vi "move_tilt_stage_simple(Sub VI).vi"() -> ()   [LabVIEW 2016]
panel:
  out "Loop idx":i32
  out "open error":errorcluster
  out "Position":i32
  out "error out":errorcluster
  in  "stop":bool
  out "DeviceKey List Out":string[](array[string])
  in  "Num repeats":i32
  out "close error":errorcluster
  in  "Relative Steps":i32
  in  "Motor":i32
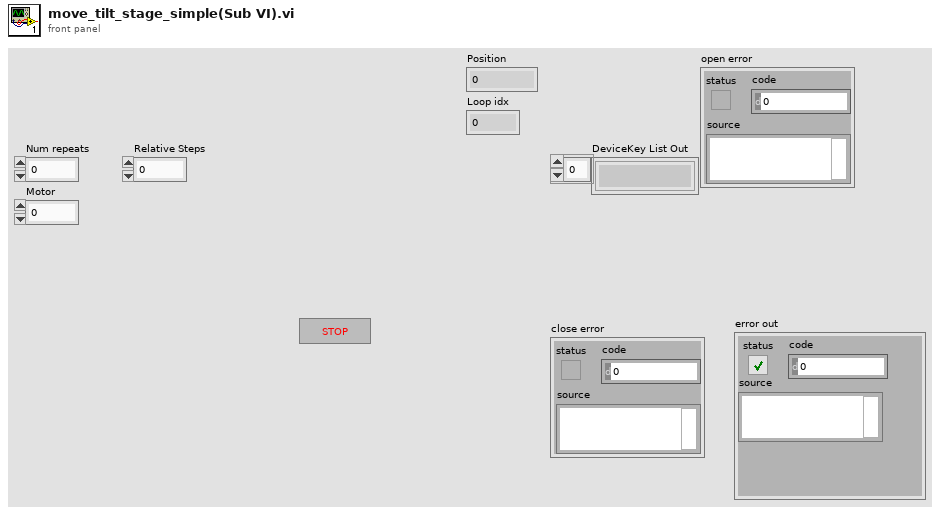
[diagram p1: front panel]
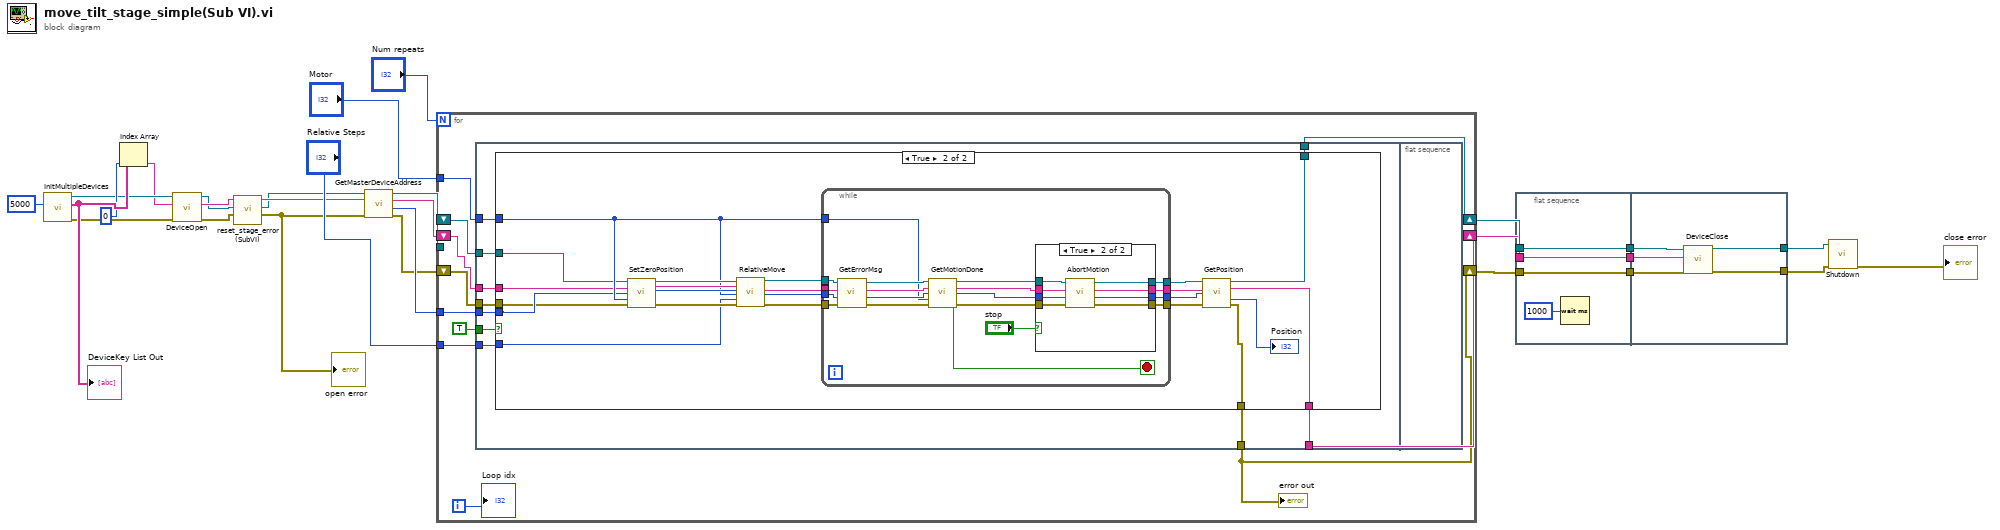
[diagram p0: block diagram]
diagram:
  n1 = call "InitMultipleDevices.vi"("msecDelayForDiscovery"=5000) -> ("error out"=w7:errorcluster, "DeviceKey List Out"=w25:string[], "CmdLib Out"=w9:refnum<k24>)  [unwired: 4 in]
  "DeviceKey List Out" <- w25
  n2 = Index Array(array=w25, index=0) -> (element=w8:string)
  n3 = call "DeviceOpen.vi"("error in (no error)"=w7, "DeviceKey In"=w8, "CmdLib In"=w9) -> ("error out"=w4:errorcluster, "DeviceKey Out"=w6:string, "CmdLib Out"=w5:refnum<k24>)  [unwired: 2 in]
  n4 = call "reset_stage_error (SubVI).vi"("error IO"=w4, "reference"=w5, "deviceKey"=w6) -> ("error IO 2"=w1:errorcluster, "new reference"=w2:refnum<k24>, "String"=w3:string)  [unwired: 6 in]
  "open error" <- w1
  n5 = call "GetMasterDeviceAddress.vi"("error in (no error)"=w1, "DeviceKey In"=w3, "CmdLib In"=w2) -> ("error out"=w19:errorcluster, "Device Address"=w20:i32, "DeviceKey Out"=w10:string, "CmdLib Out"=w21:refnum<k24>)  [unwired: 1 in]
  n6 = for {
    N: "Num repeats" -> [_]
    tunnel: "Motor" -> [w39]
    tunnel: w20 -> [w38]
    tunnel: "Relative Steps" -> [w35]
    shift-right: [w32] -> w15
    shift-left: w19 -> [w37]
    tunnel: w21 -> [_]
    shift-right: [w33] -> w16
    shift-left: w10 -> [w29]
    shift-right: [w34] -> w17
    shift-left: _ -> [w30]
    i -> [w31]
    n7 = flat-sequence {
      tunnel: w39 -> [w49]
      tunnel: w30 -> [w48]
      tunnel: w29 -> [w47]
      tunnel: [w44] -> _
      tunnel: TRUE ("Run?") -> [w46]
      tunnel: w35 -> [w45]
      tunnel: w38 -> [w44]
      tunnel: w37 -> [w43]
      tunnel: [w42] -> w34
      tunnel: [w41] -> w33
      tunnel: [w40] -> w32
      frame #0 {
        n8 = case shown="True" w46 {
          tunnel: w49 -> [_ w62]
          tunnel: w48 -> [w51 w61]
          tunnel: w47 -> [w52 w60]
          tunnel: w44 -> [_ w59]
          tunnel: w45 -> [_ w58]
          tunnel: w43 -> [w50 w57]
          tunnel: [w51 w56] -> w42
          tunnel: [w52 w55] -> w41
          tunnel: [w50 w54] -> w40
          frame False {
          }
          frame True {
            n9 = call "SetZeroPosition.vi"("CmdLib In"=w61, "DeviceKey In"=w60, "Device Address In"=w59, "Motor"=w62, "error in (no error)"=w57) -> ("CmdLib Out"=w71:refnum<k24>, "DeviceKey Out"=w70:string, "Device Address Out"=w68:i32, "error out"=w69:errorcluster)  [unwired: 7 in]
            n10 = call "RelativeMove.vi"("CmdLib In"=w71, "DeviceKey In"=w70, "Device Address In"=w68, "Motor"=w62, "Relative Steps"=w58, "error in (no error)"=w69) -> ("CmdLib Out"=w74:refnum<k24>, "DeviceKey Out"=w73:string, "Device Address Out"=w67:i32, "error out"=w72:errorcluster)  [unwired: 10 in]
            n11 = while {
              tunnel: w62 -> [w78]
              tunnel: w74 -> [w91]
              tunnel: w73 -> [w90]
              tunnel: [w86] -> w65
              tunnel: w67 -> [w85]
              tunnel: w72 -> [w89]
              tunnel: [w87] -> w66
              tunnel: [w77] -> w64
              tunnel: [w76] -> w63
              stop <- w83 stop-if-true
              n12 = call "GetErrorMsg.vi"("error in (no error)"=w89, "Device Address In"=w85, "DeviceKey In"=w90, "CmdLib In"=w91) -> ("error out"=w88:errorcluster, "Device Address Out"=w84:i32, "DeviceKey Out"=w93:string, "CmdLib Out"=w92:refnum<k24>)
              n13 = call "GetMotionDone.vi"("CmdLib In"=w92, "DeviceKey In"=w93, "Device Address In"=w84, "Motor"=w78, "error in (no error)"=w88) -> ("CmdLib Out"=w82:refnum<k24>, "DeviceKey Out"=w81:string, "Device Address Out"=w80:i32, "Is Motion Done"=w83:bool, "error out"=w79:errorcluster)  [unwired: 6 in]
              n14 = case shown="True" "stop" {
                tunnel: w79 -> [w96 w105]
                tunnel: [w96 w104] -> w87
                tunnel: w82 -> [w97 w103]
                tunnel: [w97 w102] -> w86
                tunnel: w81 -> [w94 w101]
                tunnel: w80 -> [w95 w100]
                tunnel: [w95 w99] -> w77
                tunnel: [w94 w98] -> w76
                frame False {
                }
                frame True {
                  n15 = call "AbortMotion.vi"("error in (no error)"=w105, "Device Address In"=w100, "DeviceKey In"=w101, "CmdLib In"=w103) -> ("error out"=w104:errorcluster, "Device Address Out"=w99:i32, "DeviceKey Out"=w98:string, "CmdLib Out"=w102:refnum<k24>)
                }
              }
            }
            n16 = call "GetPosition.vi"("CmdLib In"=w65, "DeviceKey In"=w63, "Device Address In"=w64, "error in (no error)"=w66) -> ("CmdLib Out"=w56:refnum<k24>, "DeviceKey Out"=w55:string, "Position"=→"Position":i32, "error out"=w54:errorcluster)  [unwired: 7 in, 1 out]
          }
        }
      }
      frame #1 {
      }
    }
    "error out" <- w32
    "Loop idx" <- w31
  }
  n17 = flat-sequence {
    tunnel: w15 -> [w107]
    tunnel: w16 -> [w108]
    tunnel: w17 -> [w109]
    tunnel: [w109] -> w28
    tunnel: [w108] -> w27
    tunnel: [w107] -> w26
    tunnel: w28 -> [w114]
    tunnel: w27 -> [w113]
    tunnel: w26 -> [w112]
    tunnel: [w111] -> w13
    tunnel: [w110] -> w11
    frame #0 {
      n18 = Wait (ms)(milliseconds to wait=u32 1000) -> ()  [unwired: 1 out]
    }
    frame #1 {
      n19 = call "DeviceClose.vi"("error in (no error)"=w112, "DeviceKey In"=w113, "CmdLib In"=w114) -> ("error out"=w111:errorcluster, "CmdLib Out"=w110:refnum<k24>)  [unwired: 2 in, 1 out]
    }
  }
  n20 = call "Shutdown.vi"("error in (no error)"=w13, "CmdLib In"=w11) -> ("error out"=→"close error":errorcluster)  [unwired: 4 in, 1 out]
